vi "GetMagnificationFromHeaderFile.vi"(8 "error in (no error)":errorcluster, 11 "File Path and Name":path=path "C:/Users/Weizmann/Desktop/LIOR/K feldspar -12_06_2014-16_45_31.txt") -> (0 "error out":errorcluster, 3 "Magnification (Microns/Pixel)":T1=2.731524 items=["5x_M_BD"=2.731524, "10x_M"=1.3634, "10xM_BD"=1.3543, "10x_ph1"=1.3439, "20x_S"=0.68129, "20x_LM"=0.714285, "50x_S"=0.277777, "100x_im"=0.119047])   [LabVIEW 2013]
doc: "Use this template to build a VI to use as a subVI."
uses:
  TypeDef/Magnification.ctl
  <vilib>/Utility/file.llb/Read From Spreadsheet File (string).vi
panel:
  out "element":string
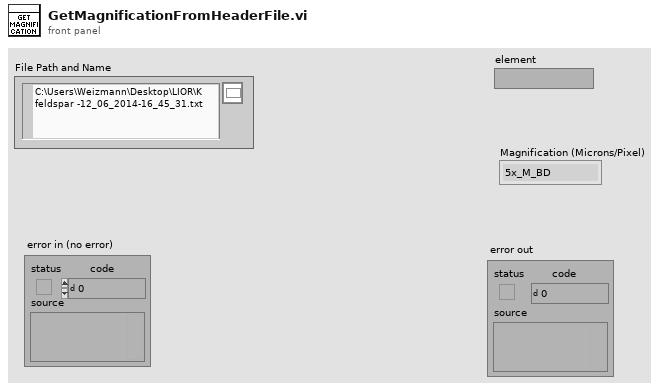
[diagram p1: front panel]
types:
  T1 = typedef "Magnification.ctl" = dbl
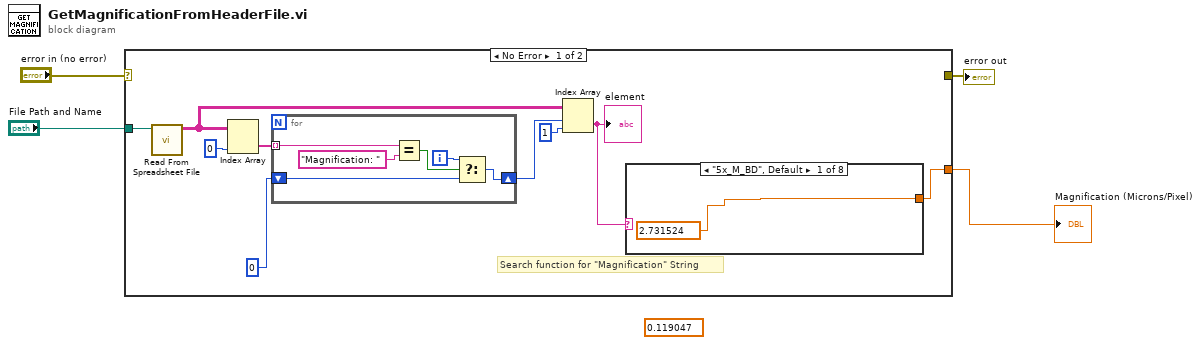
[diagram p0: block diagram]
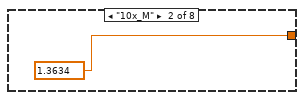
[diagram p2: hidden frame]
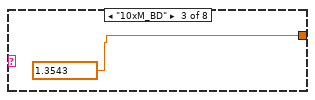
[diagram p3: hidden frame]
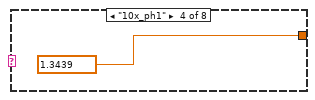
[diagram p4: hidden frame]
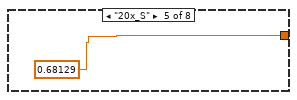
[diagram p5: hidden frame]
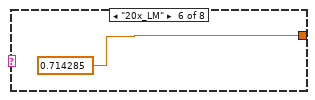
[diagram p6: hidden frame]
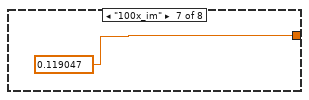
[diagram p7: hidden frame]
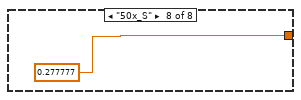
[diagram p8: hidden frame]
diagram:
  (unwired) T1 0.119047 items=["5x_M_BD"=2.731524, "10x_M"=1.3634, "10xM_BD"=1.3543, "10x_ph1"=1.3439, "20x_S"=0.68129, "20x_LM"=0.714285, "50x_S"=0.277777, "100x_im"=0.119047] ("Magnification (Microns/Pixel)")
  n1 = case shown="No Error" "error in (no error)" {
    selector: "error in (no error)" -> [_ w28]
    tunnel: [_ w28] -> w3
    tunnel: "File Path and Name" -> [w13 _]
    tunnel: [w5 _] -> w1
    frame No Error {
      # "Search function for \"Magnification\" String"
      n2 = call-poly <vilib>:"Read From Spreadsheet File.vi"("file path (dialog if empty)"=w13) -> ("all rows"=w9:string[][])  [unwired: 6 in, 4 out]
      n3 = Index Array(array=w9, index (col)=0 ("disabled index (col)")) -> (element=w11:string[])  [unwired: 1 in]
      n4 = for {
        tunnel: w11 -> [w26] mode=indexing
        shift-right: [w23] -> w8
        shift-left: 0 -> [w22]
        i -> [w24]
        n5 = Equal?(x=w26, y="Magnification: " ("string")) -> (x = y?=w25:bool)
        n6 = Select(t=w24, s=w25, f=w22) -> (s? t:f=w23:i32)
      }
      n7 = Index Array(array=w9, index (row)=w8, index (col)=1 ("disabled index (col)")) -> (element=w6:string)
      "element" <- w6
      n8 = case shown="\"5x_M_BD\", Default" w6 {
        tunnel: [w14 w15 w16 w17 w18 w19 w20 w21] -> w5
        frame "5x_M_BD", Default {
          w14 = T1 2.731524 items=["5x_M_BD"=2.731524, "10x_M"=1.3634, "10xM_BD"=1.3543, "10x_ph1"=1.3439, "20x_S"=0.68129, "20x_LM"=0.714285, "50x_S"=0.277777, "100x_im"=0.119047] ("Magnification (Microns/Pixel)")
        }
        frame "10x_M" {
          w15 = T1 1.3634 items=["5x_M_BD"=2.731524, "10x_M"=1.3634, "10xM_BD"=1.3543, "10x_ph1"=1.3439, "20x_S"=0.68129, "20x_LM"=0.714285, "50x_S"=0.277777, "100x_im"=0.119047] ("Magnification (Microns/Pixel)")
        }
        frame "10xM_BD" {
          w16 = T1 1.3543 items=["5x_M_BD"=2.731524, "10x_M"=1.3634, "10xM_BD"=1.3543, "10x_ph1"=1.3439, "20x_S"=0.68129, "20x_LM"=0.714285, "50x_S"=0.277777, "100x_im"=0.119047] ("Magnification (Microns/Pixel)")
        }
        frame "10x_ph1" {
          w17 = T1 1.3439 items=["5x_M_BD"=2.731524, "10x_M"=1.3634, "10xM_BD"=1.3543, "10x_ph1"=1.3439, "20x_S"=0.68129, "20x_LM"=0.714285, "50x_S"=0.277777, "100x_im"=0.119047] ("Magnification (Microns/Pixel)")
        }
        frame "20x_S" {
          w18 = T1 0.68129 items=["5x_M_BD"=2.731524, "10x_M"=1.3634, "10xM_BD"=1.3543, "10x_ph1"=1.3439, "20x_S"=0.68129, "20x_LM"=0.714285, "50x_S"=0.277777, "100x_im"=0.119047] ("Magnification (Microns/Pixel)")
        }
        frame "20x_LM" {
          w19 = T1 0.714285 items=["5x_M_BD"=2.731524, "10x_M"=1.3634, "10xM_BD"=1.3543, "10x_ph1"=1.3439, "20x_S"=0.68129, "20x_LM"=0.714285, "50x_S"=0.277777, "100x_im"=0.119047] ("Magnification (Microns/Pixel)")
        }
        frame "100x_im" {
          w20 = T1 0.119047 items=["5x_M_BD"=2.731524, "10x_M"=1.3634, "10xM_BD"=1.3543, "10x_ph1"=1.3439, "20x_S"=0.68129, "20x_LM"=0.714285, "50x_S"=0.277777, "100x_im"=0.119047] ("Magnification (Microns/Pixel)")
        }
        frame "50x_S" {
          w21 = T1 0.277777 items=["5x_M_BD"=2.731524, "10x_M"=1.3634, "10xM_BD"=1.3543, "10x_ph1"=1.3439, "20x_S"=0.68129, "20x_LM"=0.714285, "50x_S"=0.277777, "100x_im"=0.119047] ("Magnification (Microns/Pixel)")
        }
      }
    }
    frame Error {
    }
  }
  "error out" <- w3
  "Magnification (Microns/Pixel)" <- w1
